vi "getAllStateNames.vi"(8 "error in (no error)":errorcluster, 11 "RfOutputChannel in":refnum<class "RfOutputChannel.lvclass">) -> (0 "error out":errorcluster, 2 "state_names":string[](array[string]), 3 "RfOutputChannel out":refnum<class "RfOutputChannel.lvclass">)   [LabVIEW 2011, in "Tools.lvlib" / "DatabaseHelpers.lvlib" / "RfOutputChannel.lvclass"]
uses:
  RfOutputChannel.lvclass
  RfOutputChannel.lvclass/RfOutputChannel.ctl
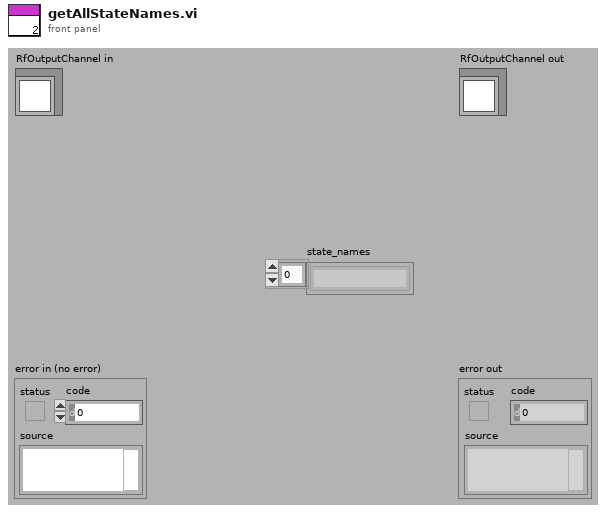
[diagram p1: front panel]
types:
  T1 = cluster{"state_name":string, "value":cluster{"frequency":string, "amplitude":string, "phase":string}}[]
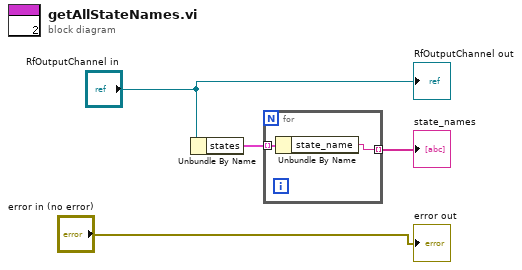
[diagram p0: block diagram]
diagram:
  n1 = Unbundle By Name("RfOutputChannel in") -> ("states"=w4:T1)
  n2 = for {
    tunnel: w4 -> [w6] mode=indexing
    tunnel: [w5] -> w3 mode=indexing
    n3 = Unbundle By Name(w6) -> ("state_name"=w5:string)
  }
  "state_names" <- w3
  "error out" <- "error in (no error)"
  "RfOutputChannel out" <- "RfOutputChannel in"
